vi "Parse RIO cal file.vi"(0 "Data In":string[][](array[string])) -> (4 "Channel Descriptions":string[][](array[string]), 6 "Cal Data":string[][](array[string]), 8 "Coefficients":string[][](array[string]), 10 "Cal Dates":string[](array[string]), 14 "As Found Data":string[][](array[string]), 15 "Verify Data":string[][](array[string]))   [LabVIEW 2013]
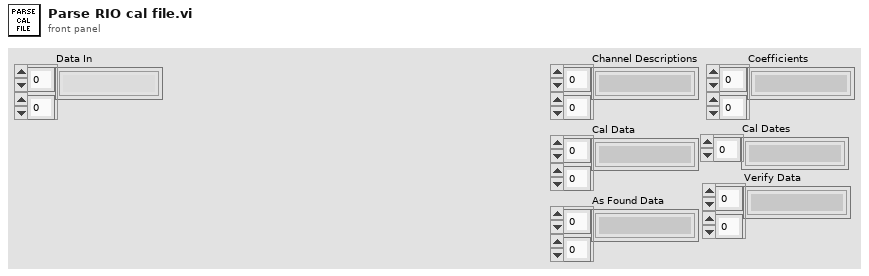
[diagram p1: front panel]
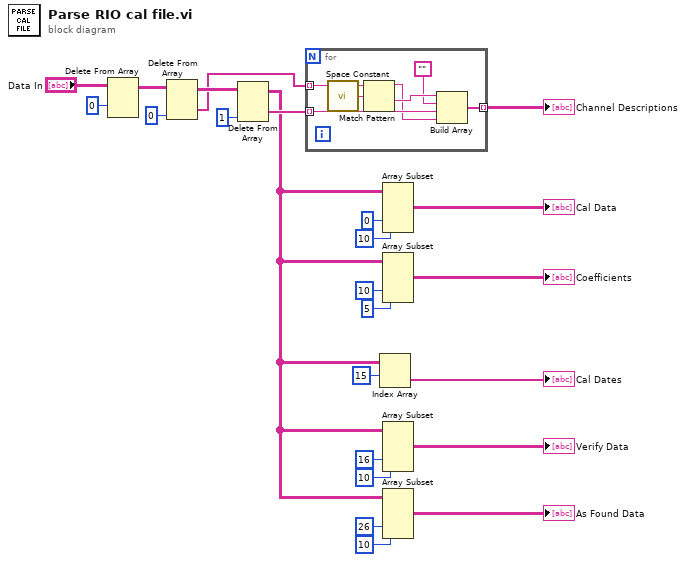
[diagram p0: block diagram]
diagram:
  n1 = Delete From Array(array="Data In", index (row)=0) -> (array with subset deleted=w18:string[][])  [unwired: 2 in, 1 out]
  n2 = Delete From Array(array=w18, index (col)=0 ("disabled index (col)")) -> (deleted portion=w16:string[], array with subset deleted=w17:string[][])  [unwired: 2 in]
  n3 = Delete From Array(array=w17, index (col)=1 ("disabled index (col)")) -> (deleted portion=w19:string[], array with subset deleted=w2:string[][])  [unwired: 2 in]
  n4 = for {
    tunnel: w16 -> [w31] mode=indexing
    tunnel: w19 -> [w28] mode=indexing
    tunnel: [w25] -> w22 mode=indexing
    n5 = call <vilib>:"Space Constant.vi"() -> ("String"=w30:string)
    n6 = Match Pattern(string=w31, regular expression=w30) -> (before substring=w27:string, after substring=w29:string)  [unwired: 1 in, 2 out]
    n7 = Build Array(w29, "", w28, w27) -> (w25:string[])
  }
  "Channel Descriptions" <- w22
  n8 = Index Array(array=w2, index (row)=15 ("index")) -> (element=→"Cal Dates":string[])  [unwired: 1 in]
  n9 = Array Subset(array=w2, index (col)=0 ("index"), length (col)=10 ("length")) -> (→"Cal Data":string[][])  [unwired: 2 in]
  n10 = Array Subset(array=w2, index (col)=10 ("index"), length (col)=5 ("length")) -> (→"Coefficients":string[][])  [unwired: 2 in]
  n11 = Array Subset(array=w2, index (col)=16 ("index"), length (col)=10 ("length")) -> (→"Verify Data":string[][])  [unwired: 2 in]
  n12 = Array Subset(array=w2, index (col)=26 ("index"), length (col)=10 ("length")) -> (→"As Found Data":string[][])  [unwired: 2 in]
